vi "Set to Array.vi"(8 "error in":errorcluster, 11 "Set":variant) -> (0 "error out":errorcluster, 3 "Array":variant)   [LabVIEW 2024, in "JSONtext.lvlib" / "SetMap.lvlib"]
uses:
  SetMap.lvlib
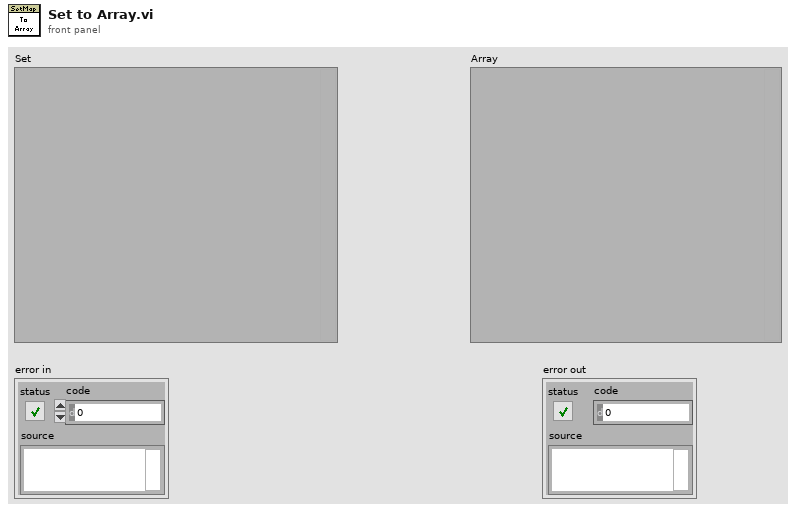
[diagram p1: front panel]
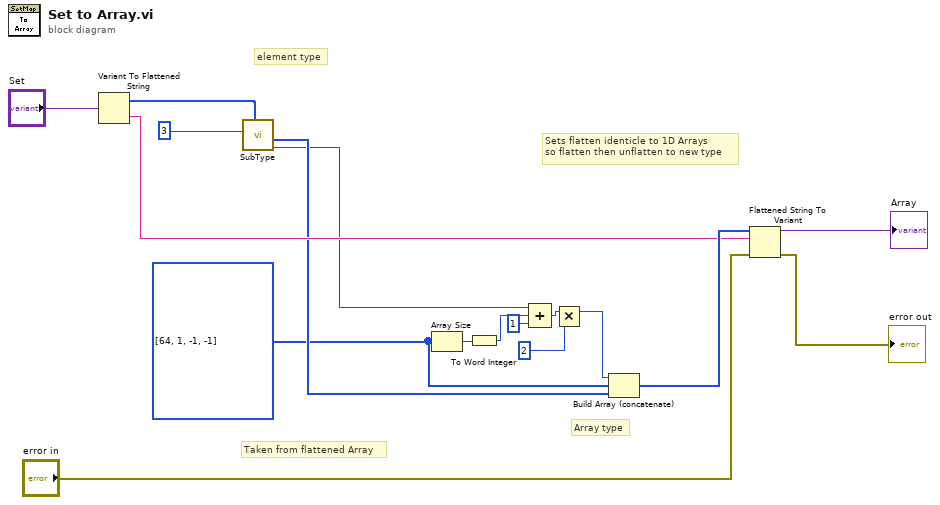
[diagram p0: block diagram]
diagram:
  w8 = i16[] [64, 1, -1, -1] ("type string 7")
  # "Taken from flattened Array"
  # "Sets flatten identicle to 1D Arrays\nso flatten then unflatten to new type"
  # "element type"
  # "Array type"
  n1 = Variant To Flattened String(Variant="Set") -> (data string=w10:string, 1:w1:i16[])
  n2 = call "SubType.vi"("type"=w1, "Offset In"=i16 3 ("index")) -> ("Size"=w2:i16, "subtype"=w9:i16[])  [unwired: 7 in, 1 out]
  n3 = Array Size(array=w8) -> (size(s)=w7:i32)
  n4 = To Word Integer(number=w7) -> (16bit integer=w5:i16)
  n5 = Compound Arithmetic op=ADD(w2, w5, i16 1 ("value")) -> (w6:i16)
  n6 = Multiply(x=w6, y=i16 2) -> (x*y=w12:i16)
  n7 = Build Array (concatenate)(w12, w8, w9) -> (w11:i16[])
  n8 = Flattened String To Variant(4:"error in", 6:w10, 7:w11) -> (0:→"error out":errorcluster, 3:→"Array":variant)
